vi "Lswitch.vi"(8 "Joy val":dbl, 10 "bottom Limit Switch":bool) -> (3 "LiftVal":dbl)   [LabVIEW 2017]
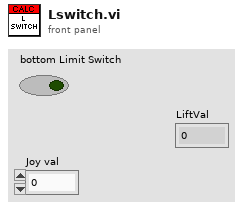
[diagram p1: front panel]
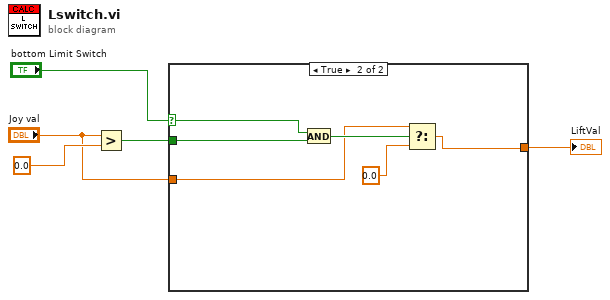
[diagram p0: block diagram]
diagram:
  n1 = Greater?(x="Joy val", y=0.0) -> (0:w1:bool)
  n2 = case shown="True" "bottom Limit Switch" {
    selector: "bottom Limit Switch" -> [_ w12]
    tunnel: "Joy val" -> [w6 w7]
    tunnel: [w6 w9] -> w3
    tunnel: w1 -> [_ w11]
    frame False {
    }
    frame True {
      n3 = And(x=w12, y=w11) -> (x .and. y?=w10:bool)
      n4 = Select(t=w7, s=w10, f=0.0 ("t")) -> (s? t:f=w9:dbl)
    }
  }
  "LiftVal" <- w3
